vi "PPS_TRAJECTORY_EXECUTE_ABS.vi"(8 "Init":bool, 11 "End Pose ENG":T7={"TRANSLATION"={"X"=0.0, "Y"=0.0}, "ROTATION"={"VALUE"=0.0, "COS"=1.0, "SIN"=0.0}} {"ROTATION"."SIN" format="%13.4f"; "ROTATION"."COS" format="%13.4f"; "ROTATION"."VALUE" format="%13.4f"; "TRANSLATION"."Y" format="%14.3f"; "TRANSLATION"."X" format="%14.3f"}) -> (0 "AtReference":bool, 3 "Chassis Velocity Target SI":T8 {"vOmega" format="%10.3f"; "vY" format="%10.3f"; "vX" format="%10.3f"})   [LabVIEW 2019]
uses:
  <vilib>/Rock Robotics/WPI/ThirdParty/JAS_Junk/TrajLib/Trajectory_Library.lvlib
  PPS_TRAJECTORY_GLOBALS.vi
  <vilib>/Rock Robotics/WPI/ThirdParty/MJansen/PathPlanner/PathPlanner24.lvlib
  <vilib>/Rock Robotics/WPI/ThirdParty/JAS_Junk/TrajLib/TypeDef/CHASSIS_SPEEDS.ctl
  <vilib>/Rock Robotics/WPI/ThirdParty/JAS_Junk/TrajLib/TypeDef/TRANSLATION2D.ctl
  <vilib>/Rock Robotics/WPI/ThirdParty/JAS_Junk/TrajLib/TypeDef/ROTATION2D.ctl
  <vilib>/Rock Robotics/WPI/ThirdParty/JAS_Junk/TrajLib/TypeDef/POSE2D.ctl
  <vilib>/Rock Robotics/WPI/ThirdParty/MJansen/PathPlanner/TypeDef/PathPlannerTrajectory.ctl
  <vilib>/Rock Robotics/WPI/ThirdParty/MJansen/PathPlanner/TypeDef/PathPlannerTrajectoryState.ctl
  <vilib>/Rock Robotics/WPI/ThirdParty/MJansen/PathPlanner/TypeDef/PathPlannerPathConstraints.ctl
panel:
  out "PathPlannerTrajectory":T1 {"States"."TargetHolonomicRotation"."SIN" format="%13.4f"; "States"."TargetHolonomicRotation"."COS" format="%13.4f"; "States"."TargetHolonomicRotation"."VALUE" format="%13.4f"; "States"."Heading"."SIN" format="%13.4f"; "States"."Heading"."COS" format="%13.4f"; "States"."Heading"."VALUE" format="%13.4f"; "States"."PositionMeters"."Y" format="%14.3f"; "States"."PositionMeters"."X" format="%14.3f"}
  in  "Robot Params":T6={"Max Module Speed M/S"=3.2, "Drive Base Radius M"=0.6}
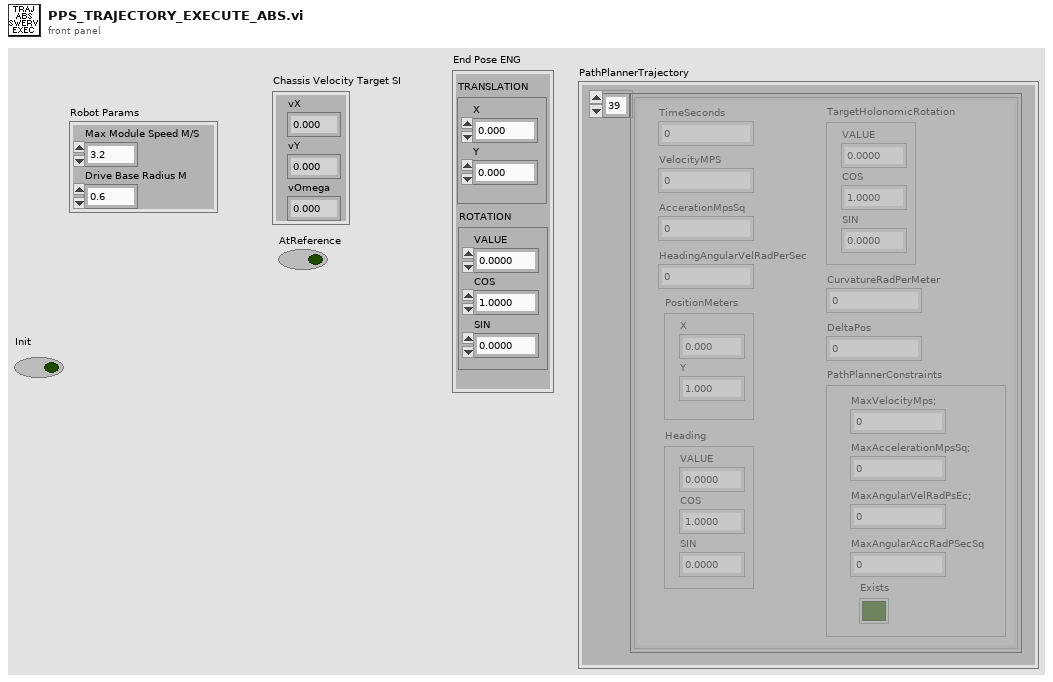
[diagram p1: front panel]
types:
  T1 = typedef "PathPlanner24.lvlib/PathPlannerTrajectory.ctl" = cluster{"States":T2[]}
  T2 = typedef "PathPlanner24.lvlib/PathPlannerTrajectoryState.ctl" = cluster{"TimeSeconds":dbl, "VelocityMPS":dbl, "AccerationMpsSq":dbl, "HeadingAngularVelRadPerSec":dbl, "PositionMeters":T3, "Heading":T4, "TargetHolonomicRotation":T4, "CurvatureRadPerMeter":dbl, "PathPlannerConstraints":T5, "DeltaPos":dbl}
  T3 = typedef "Trajectory_Library.lvlib/TRANSLATION2D.ctl" = cluster{"X":dbl, "Y":dbl}
  T4 = typedef "Trajectory_Library.lvlib/ROTATION2D.ctl" = cluster{"VALUE":dbl, "COS":dbl, "SIN":dbl}
  T5 = typedef "PathPlanner24.lvlib/PathPlannerPathConstraints.ctl" = cluster{"MaxVelocityMps;":dbl, "MaxAccelerationMpsSq;":dbl, "MaxAngularVelRadPsEc;":dbl, "MaxAngularAccRadPSecSq":dbl, "Exists":bool}
  T6 = cluster{"Max Module Speed M/S":dbl, "Drive Base Radius M":dbl}
  T7 = typedef "Trajectory_Library.lvlib/POSE2D.ctl" = cluster{"TRANSLATION":T3, "ROTATION":T4}
  T8 = typedef "Trajectory_Library.lvlib/CHASSIS_SPEEDS.ctl" = cluster{"vX":dbl, "vY":dbl, "vOmega":dbl}
  T9 = typedef "Trajectory_Library.lvlib/SWERVE_DRIVE_KINEMATICS.ctl" = cluster{"NumModules":i32, "InverseKinematics":T10, "ForwardKinematics":T10, "Modules":T3[], "PrevCoR":T3, "SavedModuleStates":T11[]}
  T10 = typedef "NI_Matrix.lvlib/RealMatrix.ctl" = dbl[][]
  T11 = typedef "Trajectory_Library.lvlib/SWERVE_DRIVE_MODULE_STATE.ctl" = cluster{"Speed":dbl, "Angle":T4}
  T12 = typedef "Trajectory_Library.lvlib/PID_TUNING.ctl" = cluster{"Kp":dbl, "Ki":dbl, "Kd":dbl, "MaximumIntegral":dbl, "MinimumIntegral":dbl}
  T13 = typedef "Trajectory_Library.lvlib/PROFILED_PID_CONTROLLER.ctl" = cluster{"Controller":T14, "Goal":T15, "Setpoint":T15, "Constraint":T16}
  T14 = typedef "Trajectory_Library.lvlib/PID_CONTROLLER.ctl" = cluster{"Kp":dbl, "Ki":dbl, "Kd":dbl, "Period":dbl, "Max_Integral":dbl, "Min_Integral":dbl, "Max_Input":dbl, "Min_Input":dbl, "Continuous":bool, "PositionError":dbl, "VelocityError":dbl, "PrevError":dbl, "TotalError":dbl, "PositionTolerance":dbl, "VelocityTolerance":dbl, "SetPoint":dbl, "Kf":dbl, "Prev_Deriv":dbl, "Prev_Deriv 2":dbl, "DerivativeFilter":bool, "Min_Output":dbl, "Max_Output":dbl, "Prev_F_P":dbl, "Prev_F_P_2":dbl, "AntiWindupActive":bool, "Measurement":dbl}
  T15 = typedef "Trajectory_Library.lvlib/TRAPEZOID_PROFILE_STATE.ctl" = cluster{"Position":dbl, "Velocity":dbl}
  T16 = typedef "Trajectory_Library.lvlib/TRAPEZOID_PROFILE_CONSTRAINT.ctl" = cluster{"MaxVelocity":dbl, "MaxAcceleration":dbl}
  T17 = typedef "Trajectory_Library.lvlib/HOLONOMIC_PACK_TUNING.ctl" = cluster{"X PID Tuning":T12, "Y PID Tuning":T12, "thetaProfiledPID_CTRL":T13}
  T18 = typedef "Trajectory_Library.lvlib/HOLONOMIC_DRV_CTRL.ctl" = cluster{"poseTolerance":T7, "poseError":T7, "Enabled":bool, "PID_xCtrl":T14, "PID_yCtrl":T14, "PROF_PID_thetaCtrl":T13, "RotationError":T4, "FirstRun":bool}
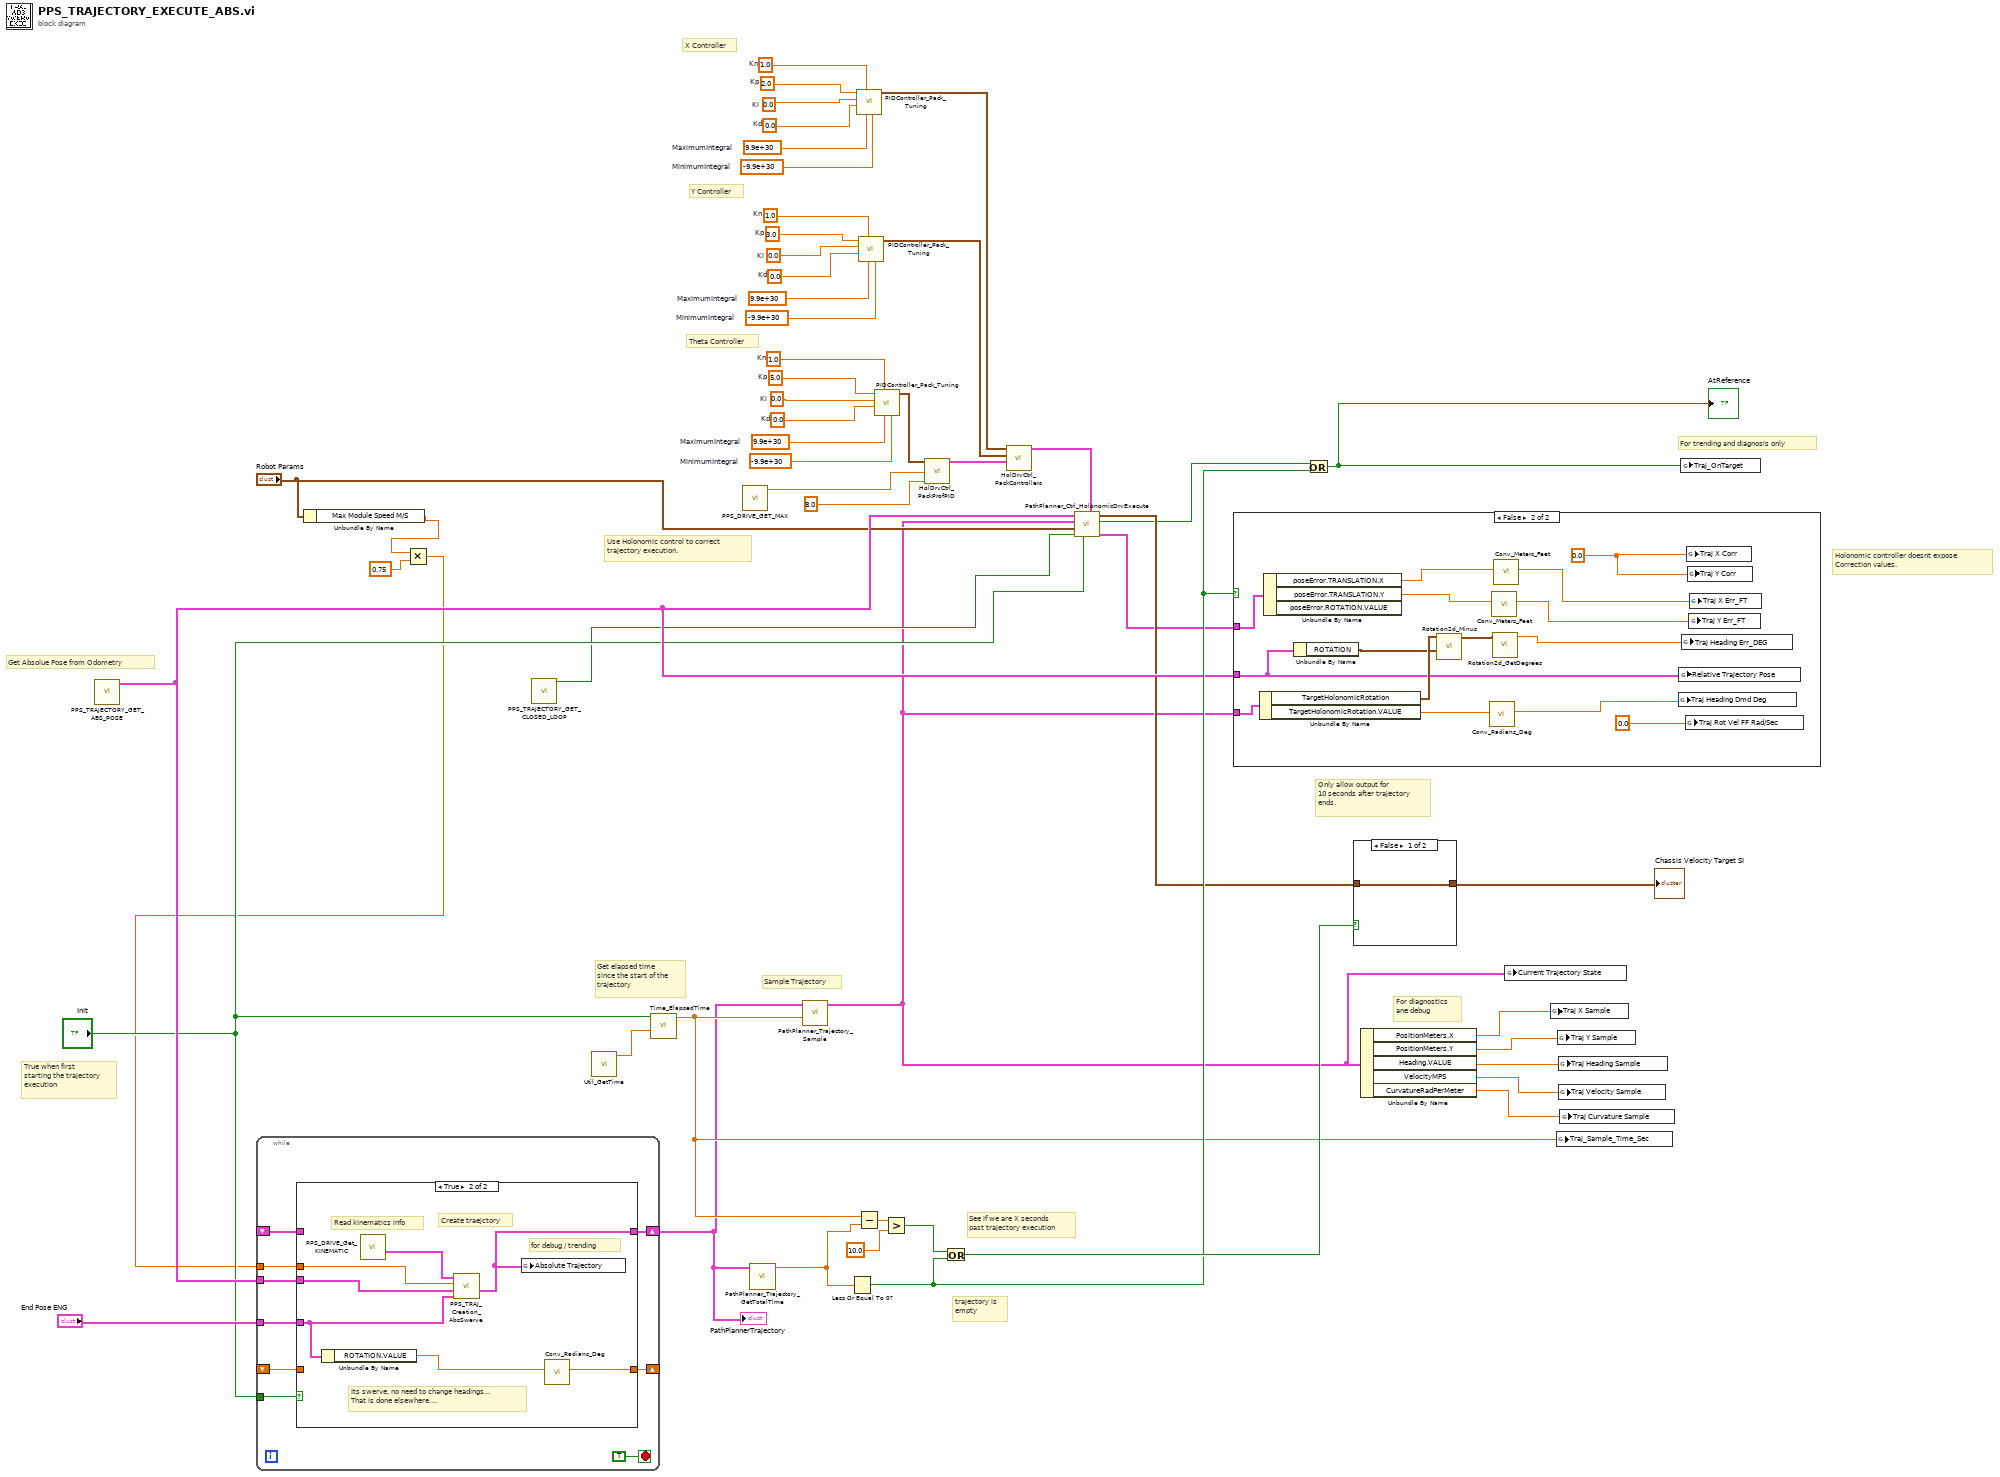
[diagram p0: block diagram]
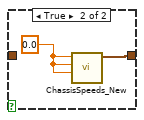
[diagram p4: hidden frame]
diagram:
  w26 = 1.0  # Kn
  w29 = 5.0  # Kp
  w38 = 0.0  # Ki
  w39 = 0.0  # Kd
  w40 = 9.9e+30  # MaximumIntegral
  w41 = -9.9e+30  # MinimumIntegral
  w24 = 1.0  # Kn
  w27 = 2.0  # Kp
  w30 = 0.0  # Ki
  w31 = 0.0  # Kd
  w32 = 9.9e+30  # MaximumIntegral
  w33 = -9.9e+30  # MinimumIntegral
  w25 = 1.0  # Kn
  w28 = 3.0  # Kp
  w34 = 0.0  # Ki
  w35 = 0.0  # Kd
  w36 = 9.9e+30  # MaximumIntegral
  w37 = -9.9e+30  # MinimumIntegral
  # "trajectory is \nempty"
  # "Theta Controller"
  # "Y Controller"
  # "X Controller"
  # "True when first\nstarting the trajectory\nexecution"
  # "Get elapsed time\nsince the start of the\ntrajectory"
  # "Holonomic controller doesnt expose\nCorrection values."
  # "Use Holonomic control to correct\ntrajectory execution."
  # "For trending and diagnosis only"
  # "For diagnostics\nane debug"
  # "Get Absolue Pose from Odometry"
  # "Sample Trajectory"
  # "See if we are X seconds \npast trajectory execution"
  # "Only allow output for\n10 seconds after trajectory\nends."
  n1 = call "PPS_TRAJECTORY_GET_ABS_POSE.vi"() -> ("Absolute Odometry Pose"=w14:T7)  [unwired: 11 in]
  n2 = Unbundle By Name("Robot Params") -> ("Max Module Speed M/S"=w2:dbl)
  n3 = Multiply(x=w2, y=0.75) -> (x*y=w3:dbl)
  n4 = while {
    tunnel: "Init" -> [w61]
    tunnel: w14 -> [w60]
    shift-right: [w59] -> w9
    shift-left: _ -> [w58]
    shift-right: [w57] -> _
    shift-left: _ -> [w56]
    tunnel: "End Pose ENG" -> [w55]
    tunnel: w3 -> [w54]
    stop <- TRUE stop-if-true
    n5 = case shown="True" w61 {
      tunnel: w60 -> [_ w66]
      tunnel: [w64 w68] -> w59
      tunnel: w58 -> [w64 _]
      tunnel: [w63 w70] -> w57
      tunnel: w56 -> [w63 _]
      tunnel: w55 -> [_ w71]
      tunnel: w54 -> [_ w65]
      frame False {
      }
      frame True {
        # "for debug / trending"
        # "Read kinematics info"
        # "Its swerve, no need to change headings...\nThat is done elsewhere...."
        # "Create traejctory"
        n6 = Unbundle By Name(w71) -> ("ROTATION.VALUE"=w69:dbl)
        n7 = call "PPS_DRIVE_Get_KINEMATIC.vi"() -> ("out SWERVE_DRIVE_KINEMATICS"=w67:T9)  [unwired: 11 in]
        n8 = call "PPS_TRAJ_Creation_AbsSwerve.vi"("End Pose  ENG"=w71, "Current Pose SI"=w66, "Max Velocity M/S"=w65, "SWERVE_DRIVE_KINEMATICS"=w67) -> ("PathPlannerTrajectory"=w68:T1)  [unwired: 5 in, 2 out]
        n9 = global write "PPS_TRAJECTORY_GLOBALS.vi" "Absolute Trajectory"(w68) -> ()
        n10 = call <vilib>:"Conv_Radians_Deg.vi"("Radians"=w69) -> ("Degrees"=w70:dbl)  [unwired: 10 in]
      }
    }
  }
  "PathPlannerTrajectory" <- w9
  n11 = call "PPS_TRAJECTORY_GET_CLOSED_LOOP.vi"() -> ("AUTO_CLOSED_LOOP"=w12:bool)  [unwired: 11 in]
  n12 = call <vilib>:"Util_GetTime.vi"() -> ("FPGA_Time_Seconds"=w50:dbl)  [unwired: 9 in, 2 out]
  n13 = call <vilib>:"Time_ElapsedTime.vi"("PassthroughTime_SEC"=w50, "Reset"="Init") -> ("Elapsed Time Sec"=w16:dbl)  [unwired: 9 in]
  n14 = call "PPS_DRIVE_GET_MAX.vi"() -> ("Max Wheel Vel (Meter/Sec)"=w4:dbl)  [unwired: 10 in, 1 out]
  n15 = call <vilib>:"PathPlanner_Trajectory_GetTotalTime.vi"("PathPlannerTrajectory"=w9) -> ("TotalTimeSeconds"=w8:dbl)  [unwired: 10 in]
  n16 = call <vilib>:"PathPlanner_Trajectory_Sample.vi"("Time"=w16, "PathPlannerTrajectory"=w9) -> ("PathPlannerState"=w5:T2)  [unwired: 9 in]
  n17 = Less Or Equal To 0?(x=w8) -> (x <= 0?=w17:bool)
  n18 = call <vilib>:"PIDController_Pack_Tuning.vi"("MinimumIntegral"=w33, "MaximumIntegral"=w32, "Kn"=w24, "Kd"=w31, "Ki"=w30, "Kp"=w27) -> ("PID Tuning"=w42:T12)  [unwired: 5 in]
  n19 = Subtract(x=w16, y=w8) -> (x-y=w53:dbl)
  n20 = call <vilib>:"PIDController_Pack_Tuning.vi"("MinimumIntegral"=w37, "MaximumIntegral"=w36, "Kn"=w25, "Kd"=w35, "Ki"=w34, "Kp"=w28) -> ("PID Tuning"=w43:T12)  [unwired: 5 in]
  n21 = call <vilib>:"PIDController_Pack_Tuning.vi"("MinimumIntegral"=w41, "MaximumIntegral"=w40, "Kn"=w26, "Kd"=w39, "Ki"=w38, "Kp"=w29) -> ("PID Tuning"=w23:T12)  [unwired: 5 in]
  n22 = Greater?(x=w53, y=10.0) -> (0:w20:bool)
  n23 = call <vilib>:"HolDrvCtrl_PackProfPID.vi"("Max Accel"=8.0, "Max Speed"=w4, "Theta PID Tuning"=w23) -> ("Theta PID CONTROLLER"=w44:T13)  [unwired: 8 in]
  n24 = Or(x=w20, y=w17) -> (x .or. y?=w19:bool)
  n25 = call <vilib>:"HolDrvCtrl_PackControllers.vi"("thetaProfiledPID_CTRL"=w44, "Y PID Tuning"=w43, "X PID Tuning"=w42) -> ("HOLONOMIC_CTRL_PACK_TUNING"=w15:T17)  [unwired: 8 in]
  n26 = call <vilib>:"PathPlanner_Ctrl_HolonomicDrvExecute.vi"("HOLONOMIC_CTRL_PACK_TUNING"=w15, "Reset"="Init", "Enabled"=w12, "Robot Parameters"="Robot Params", "PathPlannerState"=w5, "Current Pose SI"=w14) -> ("outHOLONOMIC_DRV_CTRL"=w6:T18, "At Reference"=w10:bool, "calcChassisSpeed"=w11:T8)  [unwired: 2 in, 1 out]
  n27 = case shown="False" w17 {
    tunnel: w14 -> [_ w75]
    tunnel: w6 -> [_ w82]
    tunnel: w5 -> [_ w79]
    frame True {
    }
    frame False {
      w86 = 0.0 ("Y Corr")
      n28 = Unbundle By Name(w79) -> ("TargetHolonomicRotation"=w76:T4, "TargetHolonomicRotation.VALUE"=w78:dbl)
      n29 = Unbundle By Name(w82) -> ("poseError.TRANSLATION.X"=w81:dbl, "poseError.TRANSLATION.Y"=w80:dbl)  [unwired: 1 out]
      n30 = Unbundle By Name(w75) -> ("ROTATION"=w74:T4)
      n31 = call <vilib>:"Rotation2d_Minus.vi"("other ROTATION"=w74, "in ROTATION"=w76) -> ("out ROTATION"=w73:T4)  [unwired: 9 in]
      n32 = call <vilib>:"Conv_Radians_Deg.vi"("Radians"=w78) -> ("Degrees"=w77:dbl)  [unwired: 10 in]
      n33 = call <vilib>:"Conv_Meters_Feet.vi"("Meters"=w80) -> ("Feet"=w85:dbl)  [unwired: 10 in]
      n34 = call <vilib>:"Rotation2d_GetDegrees.vi"("in ROTATION"=w73) -> ("AngleDegrees"=w72:dbl)  [unwired: 10 in]
      n35 = call <vilib>:"Conv_Meters_Feet.vi"("Meters"=w81) -> ("Feet"=w84:dbl)  [unwired: 10 in]
      n36 = global write "PPS_TRAJECTORY_GLOBALS.vi" "Traj Heading Dmd Deg"(w77) -> ()
      n37 = global write "PPS_TRAJECTORY_GLOBALS.vi" "Relative Trajectory Pose"(w75) -> ()
      n38 = global write "PPS_TRAJECTORY_GLOBALS.vi" "Traj Heading Err_DEG"(w72) -> ()
      n39 = global write "PPS_TRAJECTORY_GLOBALS.vi" "Traj Rot Vel FF Rad/Sec"(0.0 ("Traj Heading Dmd Deg")) -> ()
      n40 = global write "PPS_TRAJECTORY_GLOBALS.vi" "Traj X Corr"(w86) -> ()
      n41 = global write "PPS_TRAJECTORY_GLOBALS.vi" "Traj Y Corr"(w86) -> ()
      n42 = global write "PPS_TRAJECTORY_GLOBALS.vi" "Traj Y Err_FT"(w85) -> ()
      n43 = global write "PPS_TRAJECTORY_GLOBALS.vi" "Traj X Err_FT"(w84) -> ()
    }
  }
  n44 = Or(x=w10, y=w17) -> (x .or. y?=w18:bool)
  "AtReference" <- w18
  n45 = case shown="False" w19 {
    tunnel: w11 -> [w87 _]
    tunnel: [w87 w88] -> w51
    frame False {
    }
    frame True {
      w89 = 0.0 ("vX")
      n46 = call <vilib>:"ChassisSpeeds_New.vi"("vAngular"=w89, "vY"=w89, "vX"=w89) -> ("CHASSIS"=w88:T8)  [unwired: 8 in]
    }
  }
  "Chassis Velocity Target SI" <- w51
  n47 = Unbundle By Name(w5) -> ("PositionMeters.X"=w49:dbl, "PositionMeters.Y"=w48:dbl, "Heading.VALUE"=w47:dbl, "VelocityMPS"=w46:dbl, "CurvatureRadPerMeter"=w45:dbl)
  n48 = global write "PPS_TRAJECTORY_GLOBALS.vi" "Current Trajectory State"(w5) -> ()
  n49 = global write "PPS_TRAJECTORY_GLOBALS.vi" "Traj X Sample"(w49) -> ()
  n50 = global write "PPS_TRAJECTORY_GLOBALS.vi" "Traj_Sample_Time_Sec"(w16) -> ()
  n51 = global write "PPS_TRAJECTORY_GLOBALS.vi" "Traj Y Sample"(w48) -> ()
  n52 = global write "PPS_TRAJECTORY_GLOBALS.vi" "Traj Heading Sample"(w47) -> ()
  n53 = global write "PPS_TRAJECTORY_GLOBALS.vi" "Traj Velocity Sample"(w46) -> ()
  n54 = global write "PPS_TRAJECTORY_GLOBALS.vi" "Traj Curvature Sample"(w45) -> ()
  n55 = global write "PPS_TRAJECTORY_GLOBALS.vi" "Traj_OnTarget"(w18) -> ()
